vi "Target to Host - Host.vi"() -> ()   [LabVIEW 2010]
uses:
  <vilib>/userDefined/High Color/nirio_resource_hc.ctl
  <vilib>/rvi/interface/nirviOpenFPGA/nirviOpenFPGA.xnode
  Target to Host - FPGA.vi
  <vilib>/rvi/interface/nirviOpenFPGA/nirviOpenFPGA.ctl
  <vilib>/rvi/interface/nirviOpenFPGA/nirviopenstate.ctl
  <vilib>/picture/picture.llb/imagedata.ctl
  <vilib>/rvi/interface/common/nirviIntfCommonState.ctl
  <vilib>/rvi/interface/common/nirviIntfModes.ctl
  Program Files/National Instruments/LabVIEW 2010/resource/RVI/emulation/niLvFpgaEmulationMode.ctl
  <vilib>/eio/XNode/Errors/EIOXNodeErrorStruct.ctl
  <vilib>/eio/XNode/Errors/EIOXNodeInternalErrorTypes.ctl
  <vilib>/eio/XNode/Errors/EIOXNodeUserErrorTypes.ctl
  <vilib>/XNodeSupport/XNodeRect32.ctl
  <vilib>/XNodeSupport/XNodeInt.ctl
  <vilib>/XNodeSupport/XNodeTerms.ctl
  <vilib>/XNodeSupport/XNodeTerm.ctl
  <vilib>/XNodeSupport/XNodeString.ctl
  <vilib>/XNodeSupport/XNodeVariant.ctl
  <vilib>/XNodeSupport/XNodeBool.ctl
  <vilib>/rvi/interface/nirviMethod/nirviMethod.xnode
  <vilib>/rvi/interface/common/niFpgaNodeNameForErrorReporting.ctl
  <vilib>/rvi/interface/nirviCloseFPGA/nirviCloseFPGA.xnode
  <vilib>/rvi/interface/RandomDataEmulation/nirviRandomDataOpen.vi
  <vilib>/rvi/interface/RandomDataEmulation/nirviRandomDataRunMethod.vi
  <vilib>/rvi/interface/RandomDataEmulation/nirviRandomDataWaitOnIRQMethod.vi
  <vilib>/rvi/interface/RandomDataEmulation/nirviRandomDataAcknowledgeIRQMethod.vi
  <vilib>/rvi/interface/RandomDataEmulation/nirviRandomDataDMAMethods.vi
  <vilib>/rvi/interface/RandomDataEmulation/nirviRandomDataClose.vi
  <vilib>/XNodeSupport/NI_XNodeSupport.lvlib
panel:
  in  "Read Period (msec)":u32=500
  out "Writing":bool
  out "Reading":bool
  out "Target to Host FIFO":u32(slide) step=416361304 scale=0.0..15.0
  in  "Stop":bool
  in  "Write Period(mSec)":u32=250
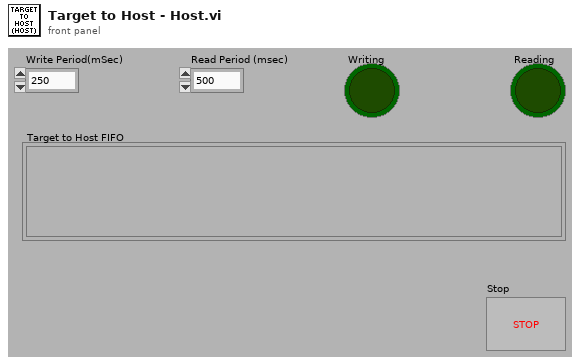
[diagram p1: front panel]
types:
  T1 = typedef "niFpgaNodeNameForErrorReporting.ctl" = enum16{"Open FPGA VI Reference", "Read/Write Control", "Invoke Method: Abort", "Invoke Method: Acknowledge IRQ", "Invoke Method: Download", "Invoke Method: FIFO.Configure", "Invoke Method: FIFO.Read", "Invoke Method: FIFO.Start", "Invoke Method: FIFO.Stop", "Invoke Method: FIFO.Write", "Invoke Method: Reset", "Invoke Method: Run", "Invoke Method: Wait on IRQ", "Close FPGA VI Reference"}
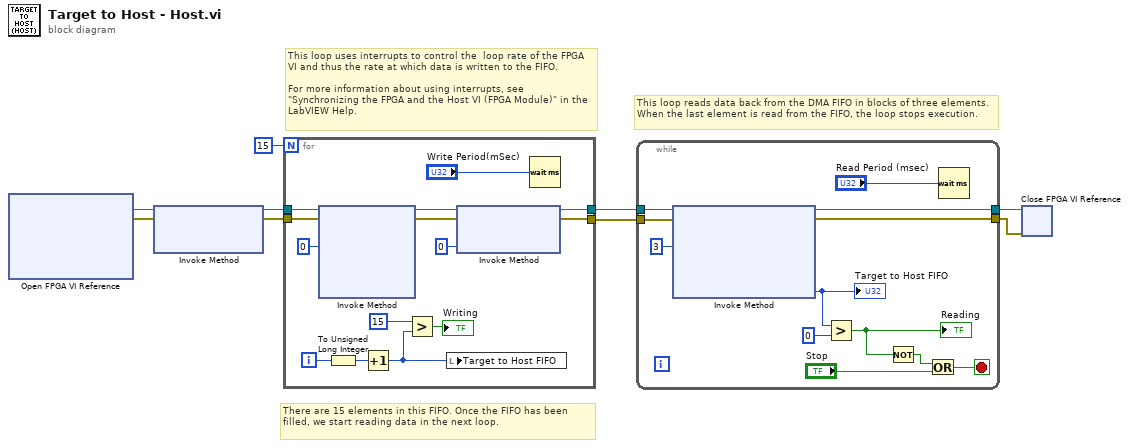
[diagram p0: block diagram]
diagram:
  # "There are 15 elements in this FIFO. Once the FIFO has been filled, we start reading data in the next loop."
  # "This loop reads data back from the DMA FIFO in blocks of three elements.  When the last element is read from the FIFO, the loop stops execution."
  # "This loop uses interrupts to control the  loop rate of the FPGA VI and thus the rate at which data is written to the FIFO.\n\nFor more information about using interrupts, see \"Synchronizing the FPGA and the Host VI (FPGA Module)\" in the LabVIEW Help."
  n1 = xnode "Open FPGA VI Reference"() -> ("FPGA VI Reference Out"=w2:refnum<k20>, "error out"=w1:errorcluster)  [unwired: 2 in]
  n2 = xnode "Invoke Method"("FPGA VI Reference In"=w2, "error in"=w1) -> ("FPGA VI Reference Out"=w9:refnum<k20>, "error out"=w8:errorcluster)  [unwired: 1 in]
  n3 = for {
    N: 15 -> [_]
    tunnel: w9 -> [w23]
    tunnel: w8 -> [w22]
    tunnel: [w14] -> w7
    tunnel: [w13] -> w6
    i -> [w17]
    n4 = xnode "Invoke Method"("FPGA VI Reference In"=w23, "error in"=w22, "IRQ Number(s)"=0) -> ("FPGA VI Reference Out"=w21:refnum<k20>, "error out"=w20:errorcluster)  [unwired: 1 in, 2 out]
    n5 = To Unsigned Long Integer(number=w17) -> (unsigned 32bit integer=w16:u32)
    n6 = Increment(x=w16) -> (x+1=w10:u32)
    n7 = Greater?(x=u32 15 ("y"), y=w10) -> (0:→"Writing":bool)
    n8 = local write "Target to Host FIFO"(w10) -> ()
    n9 = xnode "Invoke Method"("FPGA VI Reference In"=w21, "error in"=w20, "IRQ Number(s)"=0) -> ("FPGA VI Reference Out"=w14:refnum<k20>, "error out"=w13:errorcluster)
    n10 = Wait (ms)(milliseconds to wait="Write Period(mSec)") -> ()  [unwired: 1 out]
  }
  n11 = while {
    tunnel: w7 -> [w52]
    tunnel: w6 -> [w51]
    tunnel: [w50] -> w5
    tunnel: [w49] -> w4
    stop <- w45 stop-if-true
    n12 = xnode "Invoke Method"("FPGA VI Reference In"=w52, "error in"=w51, "Number of Elements"=u32 3 ("x")) -> ("FPGA VI Reference Out"=w50:refnum<k20>, "error out"=w49:errorcluster, "Elements Remaining"=w46:u32)  [unwired: 1 in, 1 out]
    "Target to Host FIFO" <- w46
    n13 = Greater?(x=w46, y=u32 0) -> (0:w42:bool)
    "Reading" <- w42
    n14 = Not(x=w42) -> (.not. x?=w43:bool)
    n15 = Or(x=w43, y="Stop") -> (x .or. y?=w45:bool)
    n16 = Wait (ms)(milliseconds to wait="Read Period (msec)") -> ()  [unwired: 1 out]
  }
  n17 = xnode "Close FPGA VI Reference"("FPGA VI Reference In"=w5, "error in"=w4) -> ()  [unwired: 1 out]
